vi "config_timebase_OSC_working.vi"(8 "error in (no error)":errorcluster, 9 "resolution":i32=10000 caption="Record Length (10000s)", 10 "hor scale":dbl, 11 "VISA resource name":refnum<visa-resource-name>) -> (0 "error out":errorcluster, 1 "concatenated string":string, 3 "VISA resource name out":refnum<visa-resource-name>)   [LabVIEW 2011]
doc: "Configures the timebase and horizontal properties of an oscilloscope."
panel:
  in  "Record Length (10000)":i32=10000 caption="Record Length (10000s)"
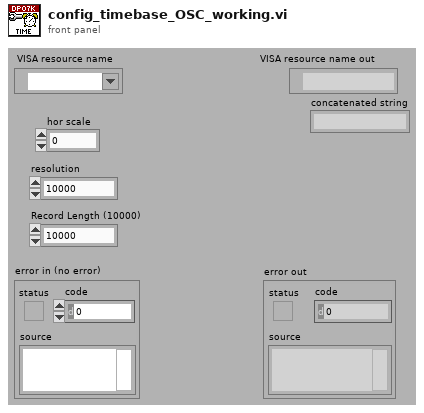
[diagram p1: front panel]
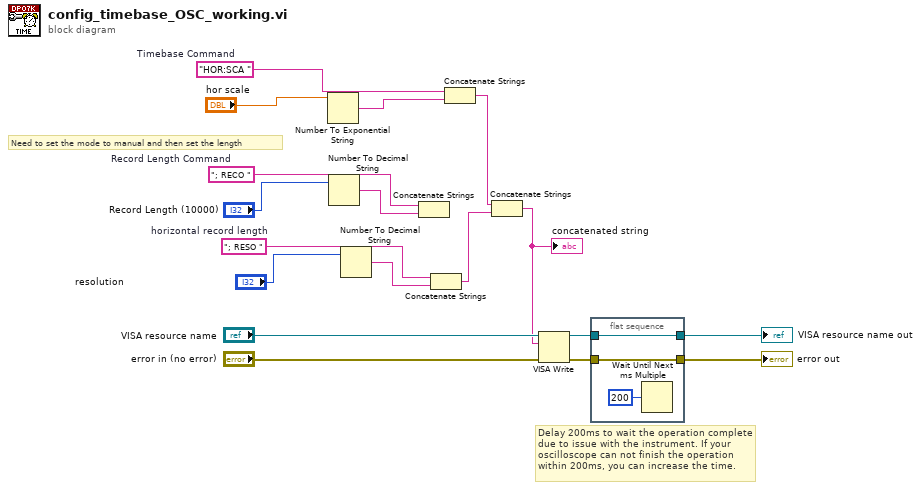
[diagram p0: block diagram]
diagram:
  w5 = "; RESO "  # horizontal record length
  w8 = "; RECO "  # Record Length Command
  w12 = "HOR:SCA "  # Timebase Command
  # "Need to set the mode to manual and then set the length"
  # "Delay 200ms to wait the operation complete due to issue with the instrument. If your oscilloscope can not finish the operation within 200ms, you can increase the time."
  n1 = Number To Exponential String(number="hor scale") -> (E-format string=w11:string)  [unwired: 3 in]
  n2 = Number To Decimal String(number="Record Length (10000)") -> (decimal integer string=w7:string)  [unwired: 1 in]
  n3 = Number To Decimal String(number="resolution") -> (decimal integer string=w4:string)  [unwired: 1 in]
  n4 = Concatenate Strings(w8, w7) -> ()  [unwired: 1 out]
  n5 = Concatenate Strings(w5, w4) -> (w3:string)
  n6 = Concatenate Strings(w12, w11) -> (w2:string)
  n7 = Concatenate Strings(w2, w3) -> (w1:string)
  "concatenated string" <- w1
  n8 = VISA Write(VISA resource name="VISA resource name", write buffer=w1, error in (no error)="error in (no error)") -> (VISA resource name out=w17:refnum<visa-resource-name>, error out=w16:errorcluster)  [unwired: 1 out]
  n9 = flat-sequence {
    tunnel: w17 -> [w20]
    tunnel: [w20] -> w14
    tunnel: w16 -> [w19]
    tunnel: [w19] -> w13
    frame #0 {
      n10 = Wait Until Next ms Multiple(millisecond multiple=u32 200) -> ()  [unwired: 1 out]
    }
  }
  "VISA resource name out" <- w14
  "error out" <- w13
